vi "short.vi"(8 "error in (no error)":errorcluster, 11 "VISA resource name":refnum<visa-resource-name>) -> (0 "error out":errorcluster, 1 "X":dbl, 2 "R":dbl, 3 "VISA resource name out":refnum<visa-resource-name>)   [LabVIEW 2016]
panel:
  in  "Enable Short Correction (F: Disable)":bool
  in  "Short Supplementary Threshold (0)":dbl
  in  "Short Capacitance Threshold (0)":dbl
  in  "Short Correction Type (0: Resistance- Reactance)":u16(ring) items=[" Resistance- Reactance", "Series Inductance- Series Resistance"]
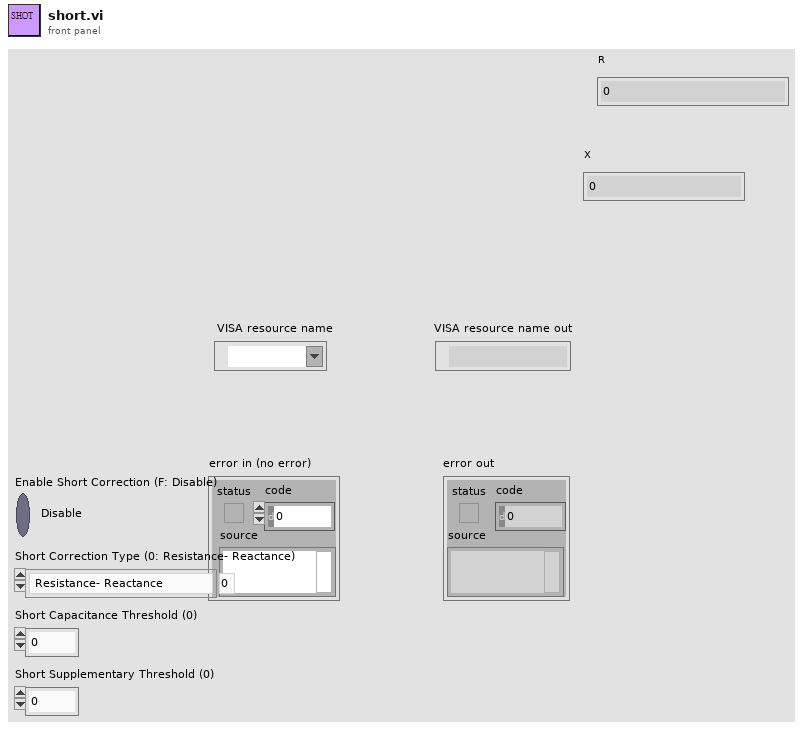
[diagram p1: front panel]
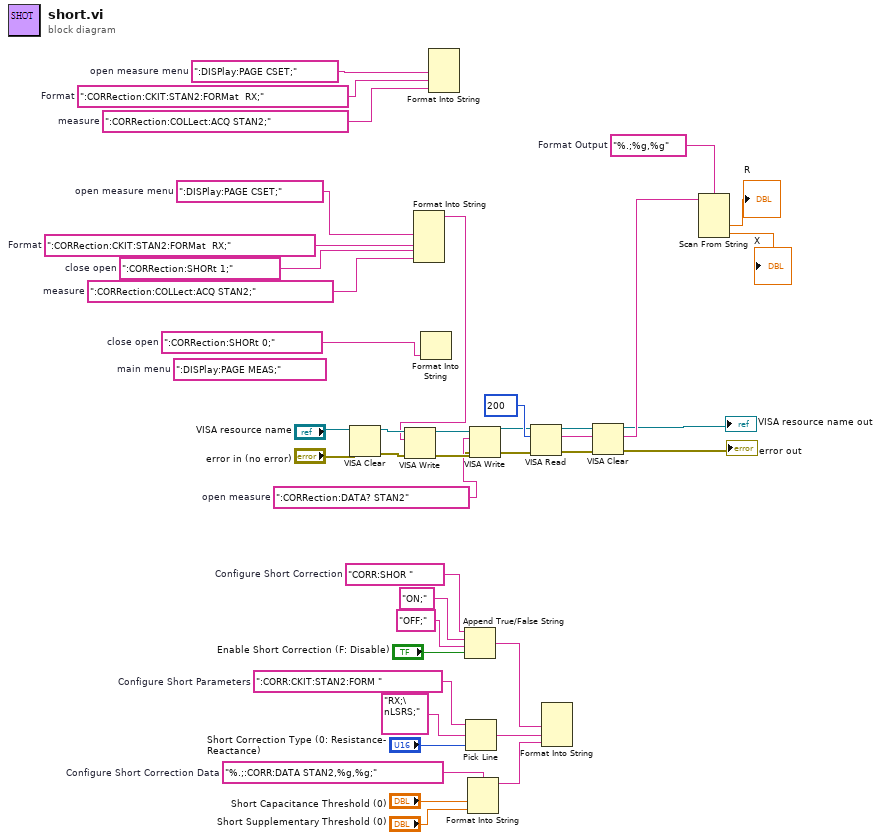
[diagram p0: block diagram]
diagram:
  w2 = ":CORRection:SHORt 1;"  # close open
  w6 = ":CORRection:COLLect:ACQ STAN2;"  # measure
  w5 = ":CORRection:CKIT:STAN2:FORMat  RX;"  # Format
  w4 = ":DISPlay:PAGE CSET;"  # open measure menu
  w12 = "%.;%g,%g"  # Format Output
  w19 = ":CORRection:DATA? STAN2"  # open measure
  w26 = ":CORRection:SHORt 0;"  # close open
  w27 = ":CORRection:COLLect:ACQ STAN2;"  # measure
  w1 = ":CORRection:CKIT:STAN2:FORMat  RX;"  # Format
  (unwired) ":DISPlay:PAGE MEAS;"  # main menu
  w3 = ":DISPlay:PAGE CSET;"  # open measure menu
  w32 = "%.;:CORR:DATA STAN2,%g,%g;"  # Configure Short Correction Data
  w36 = ":CORR:CKIT:STAN2:FORM "  # Configure Short Parameters
  w40 = "CORR:SHOR "  # Configure Short Correction
  n1 = VISA Clear(VISA resource name="VISA resource name", error in (no error)="error in (no error)") -> (VISA resource name out=w25:refnum<visa-resource-name>, error out=w24:errorcluster)
  n2 = Format Into String(w3, w1, w2, w27) -> (resulting string=w15:string)  [unwired: 3 in, 1 out]
  n3 = VISA Write(VISA resource name=w25, write buffer=w15, error in (no error)=w24) -> (VISA resource name out=w21:refnum<visa-resource-name>, error out=w20:errorcluster)  [unwired: 1 out]
  n4 = Format Into String(w26) -> ()  [unwired: 3 in, 2 out]
  n5 = Format Into String(w4, w5, w6) -> ()  [unwired: 3 in, 2 out]
  n6 = Append True/False String(1:"Enable Short Correction (F: Disable)", 2:"OFF;" ("true string"), 3:"ON;" ("true string"), 4:w40) -> (0:w29:string)
  n7 = Pick Line(string ("")=w36, multi-line string="RX;\nLSRS;", line index="Short Correction Type (0: Resistance- Reactance)") -> (output string=w30:string)
  n8 = Format Into String(format string=w32, "Short Capacitance Threshold (0)", "Short Supplementary Threshold (0)") -> (resulting string=w28:string)  [unwired: 2 in, 1 out]
  n9 = VISA Write(VISA resource name=w21, write buffer=w19, error in (no error)=w20) -> (VISA resource name out=w16:refnum<visa-resource-name>, error out=w17:errorcluster)  [unwired: 1 out]
  n10 = VISA Read(VISA resource name=w16, byte count=u32 200, error in (no error)=w17) -> (VISA resource name out=w10:refnum<visa-resource-name>, read buffer=w11:string, error out=w9:errorcluster)  [unwired: 1 out]
  n11 = Format Into String(w29, w30, w28) -> ()  [unwired: 3 in, 2 out]
  n12 = VISA Clear(VISA resource name=w10, error in (no error)=w9) -> (VISA resource name out=→"VISA resource name out":refnum<visa-resource-name>, error out=→"error out":errorcluster)
  n13 = Scan From String(format string=w12, input string=w11) -> (output 1=→"R":dbl, output 2=→"X":dbl)  [unwired: 4 in, 3 out]
